vi "运维调试_采配水.vi"() -> ()   [LabVIEW 2016, in "PLC.lvlib"]
uses:
  PLC.lvlib
  <vilib>/Plasmionique/MB Master/MB_Master/MB_Master.lvclass
  <vilib>/Utility/miscctls.llb/LVPointTypeDef.ctl
  <vilib>/Plasmionique/MB Master/MB_Master_Serial/MB_Master_Serial.lvclass
  F:/Program Files/National Instruments/LabVIEW 2016/vi.lib/Plasmionique/MB Master/MB_Master/MB_Master.lvclass
  <vilib>/Plasmionique/MB Master/MB Master.lvlib
panel:
  out "R111":i16 caption="排液时间"
  out "R22":i16
  in  "V8":bool
  out "通讯故障指示":bool
  out "R21":i16
  in  "V7":bool
  out "R20":i16
  in  "M1-2":bool
  in  "潜水泵工作模式":u16(ring) items=["泵1单泵单管路", "泵2单泵单管路", "双泵双管路"]
  out "X10":bool caption="废液报警"
  out "X9":bool caption="自来水报警"
  out "X8":bool caption="泵2过载报警"
  out "X7":bool caption="泵1过载报警"
  out "X6":bool caption="断电检测"
  out "X5":bool caption="开门检测"
  out "X4":bool caption="烟雾检测"
  out "X3":bool caption="漏水检测"
  out "X2":bool caption="进样检测"
  out "X1":bool
  out "X0":bool caption="采样池液位开关"
  out "Y12":bool caption="多参通电"
  out "R109":i16 caption="配水时间"
  out "集成报警信息":string
  out "R108":i16 caption="自来水报警"
  out "R107":i16 caption="采水池液位报警设置"
  out "R106":i16 caption="进样超时设置"
  out "R105":i16 caption="二级清洗时间"
  out "R104":i16 caption="一级清洗时间"
  out "R103":i16 caption="外部管路清洗时间"
  out "R102":i16 caption="静置沉淀时间"
  out "R101":i16 caption="内部管路润洗时间"
  out "R100":i16 caption="外部管路润洗时间"
  out "R2":i16
  out "R1":i16
  out "多列列表框":i32(listbox)
  out "R19":i16
  in  "V6":bool
  out "R18":i16
  in  "V5":bool
  out "R17":i16
  in  "V4":bool
  out "R16":i16
  in  "V3":bool
  out "R15":i16
  in  "V2":bool
  out "R14":i16
  in  "M2":bool
  out "R13":i16
  in  "V1":bool
  out "R12":i16
  in  "M1-1":bool
  in  "返回":bool
  in  "参数设置":bool
  in  "单步启动":bool
  in  "启动":bool
  in  "停止":bool
  # "S"
  # "S"
  # "S"
  # "S"
  # "S"
  # "S"
  # "S"
  # "S"
  # "S"
  # "S"
  # "S"
  # "单步计时："
  # "s"
  # "流程计时："
  # "s"
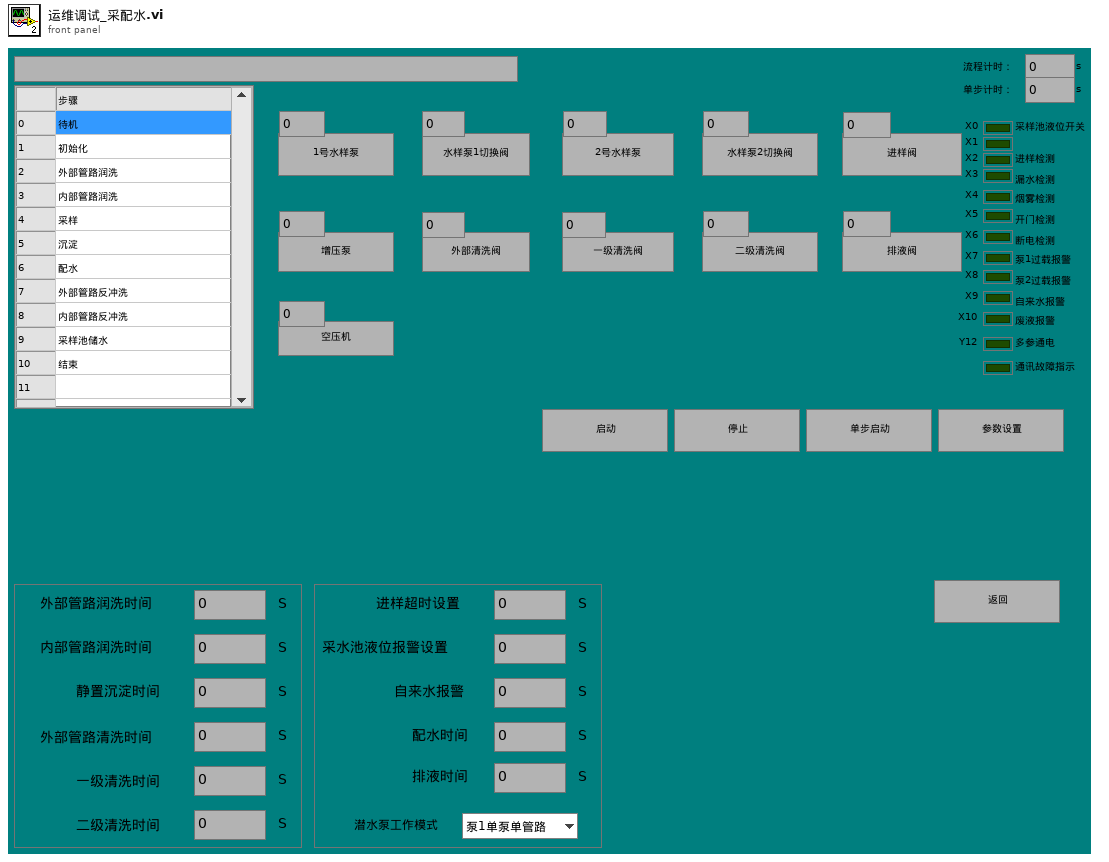
[diagram p1: front panel]
types:
  T1 = typedef "LVPointTypeDef.ctl" = cluster{"Horizontal":i16, "Vertical":i16}
  T2 = cluster{"时间标识":timestamp, "设备":string, "日志信息":string}
  T3 = cluster{"R0":i16, "R1":i16, "R2":i16, "R3":i16, "R4":i16, "R5":i16, "R6":i16, "R7":i16, "R8":i16, "R9":i16, "R10":i16, "R11":i16, "R12":i16, "R13":i16, "R14":i16, "R15":i16, "R16":i16, "R17":i16, "R18":i16, "R19":i16, "R20":i16, "R21":i16, "R22":i16}
  T4 = cluster{"coil values[0]":bool, "coil values[1]":bool, "coil values[2]":bool, "coil values[3]":bool, "coil values[4]":bool, "coil values[5]":bool, "coil values[6]":bool, "coil values[7]":bool, "coil values[8]":bool, "coil values[9]":bool, "coil values[10]":bool, "coil values[11]":bool, "coil values[12]":bool, "coil values[13]":bool, "coil values[14]":bool, "coil values[15]":bool}
  T5 = cluster{"seconds since 1Jan1904":timestamp, "table输入":string, string, "table输入":string}
  T6 = cluster{"时间标识":timestamp, "设备":string, "日志信息":string, "流程参数":string}
  T7 = cluster{"命令":string, cluster{"starting address":u16, "holding register value":u16}}
  T8 = cluster{"CODMn":cluster{"启动测量模式":cluster{"测量模式":enum16{"水样测量", "标样核查", "零点核查", "加标回收", "平行样", "校零", "校标"}}, "确定按钮":bool}, "参数启用":cluster{"多参数":bool, "CODMn":bool, "总磷总氮":bool, "氨氮":bool, "CODcr":bool}}
  T9 = enum16{"水样测量", "标样核查", "零点核查", "加标回收", "平行样", "校零", "校标"}
  T10 = cluster{"命令":string, "数据":cluster{"starting address":u16, "holding register value":u16}}
  T11 = cluster{"命令":string, "数据":cluster{"starting address":u16, "holding register values":u16[]}}
  T12 = cluster{"命令":string, "data":cluster{"starting address":u16, "coil values":bool[]}}
  T13 = enum32{"Bad", "Idle", "Run top level", "Running"}
  T14 = cluster{"baud rate (bps)":u32, "stop bits":u16, "parity":u16, "flow control":u16, "timeout":u32, "retries":i32}
  T15 = cluster{"starting address":u16, "holding register values":u16[]}
  T16 = cluster{"starting address":u16, "holding register value":u16}
  T17 = cluster{"starting address":u16, "coil values":bool[]}
  T18 = cluster{"Registers[0]":u16, "Registers[1]":u16, "Registers[2]":u16, "Registers[3]":u16, "Registers[4]":u16, "Registers[5]":u16, "Registers[6]":u16, "Registers[7]":u16, "Registers[8]":u16, "Registers[9]":u16, "Registers[10]":u16, "Registers[11]":u16, "Registers[12]":u16, "Registers[13]":u16, "Registers[14]":u16, "Registers[15]":u16, "Registers[16]":u16, "Registers[17]":u16, "Registers[18]":u16, "Registers[19]":u16, "Registers[20]":u16, "Registers[21]":u16, "Registers[22]":u16}
  T19 = cluster{"Registers[0]":u16, "Registers[1]":u16, "Registers[2]":u16, "Registers[3]":u16, "Registers[4]":u16, "Registers[5]":u16}
  T20 = cluster{"Coils[0]":bool, "Coils[1]":bool, "Coils[2]":bool, "Coils[3]":bool, "Coils[4]":bool, "Coils[5]":bool, "Coils[6]":bool, "Coils[7]":bool, "Coils[8]":bool, "Coils[9]":bool, "Coils[10]":bool, "Coils[11]":bool, "Coils[12]":bool, "Coils[13]":bool, "Coils[14]":bool, "Coils[15]":bool}
  T21 = cluster{"Registers[0]":u16, "Registers[1]":u16, "Registers[2]":u16, "Registers[3]":u16, "Registers[4]":u16, "Registers[5]":u16, "Registers[6]":u16, "Registers[7]":u16, "Registers[8]":u16, "Registers[9]":u16, "Registers[10]":u16, "Registers[11]":u16, "Registers[12]":u16, "Registers[13]":u16, "Registers[14]":u16, "Registers[15]":u16, "Registers[16]":u16, "Registers[17]":u16, "Registers[18]":u16, "Registers[19]":u16}
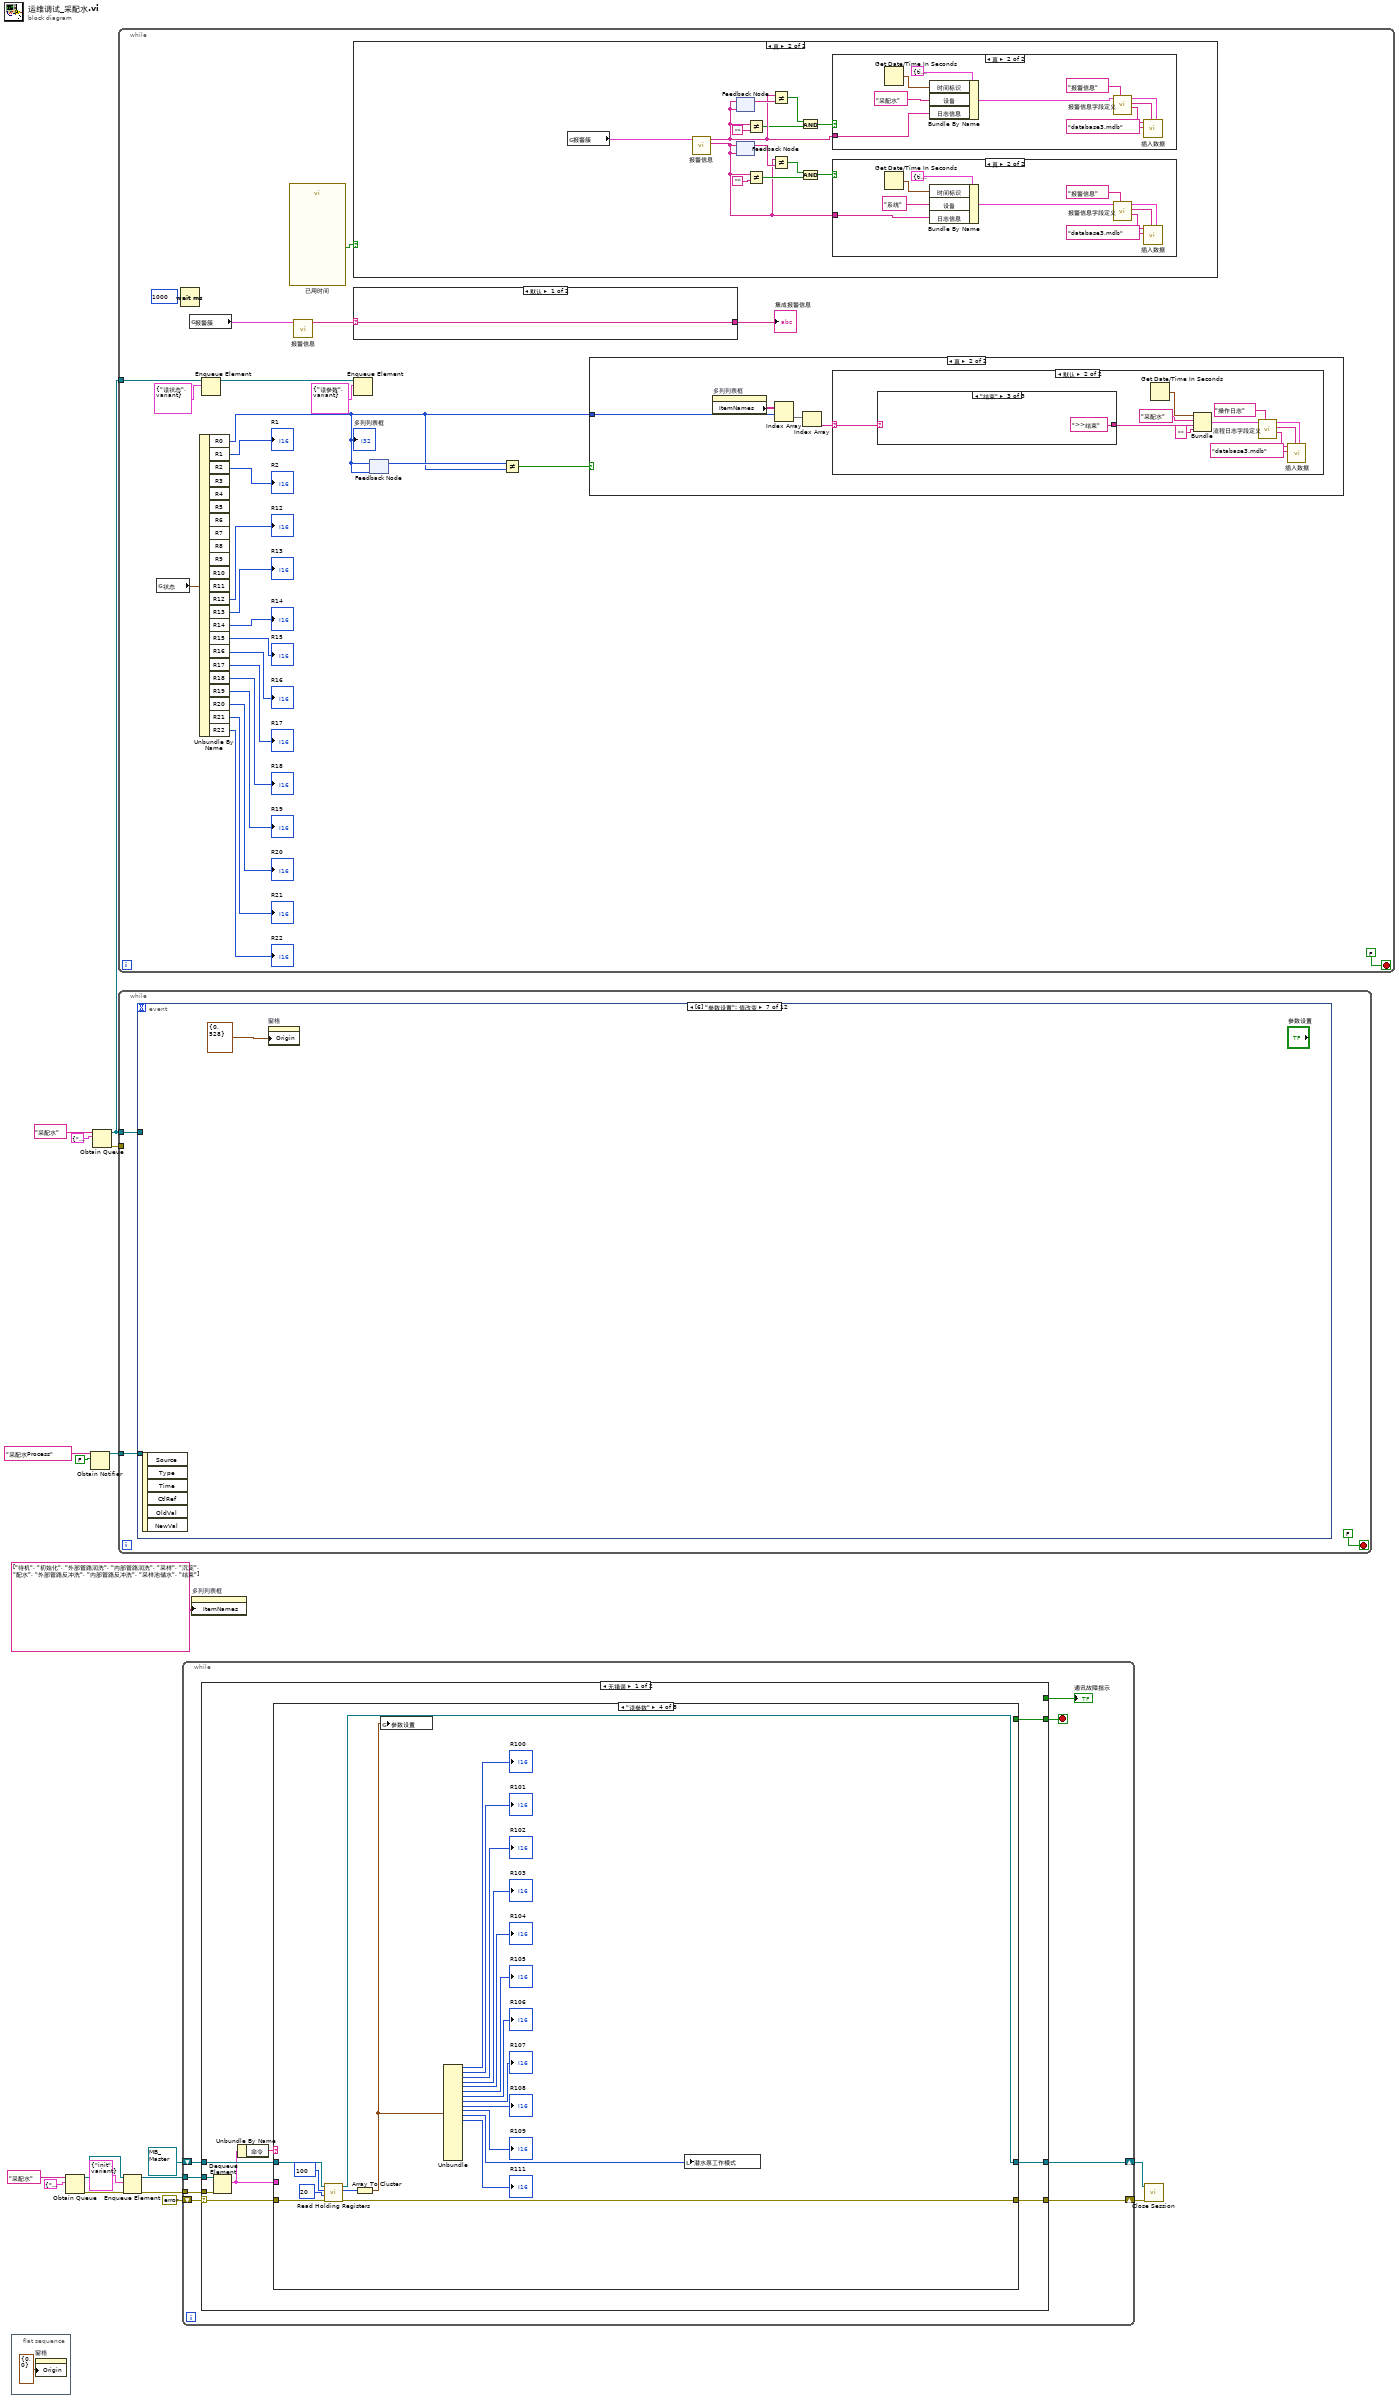
[diagram p0: block diagram]
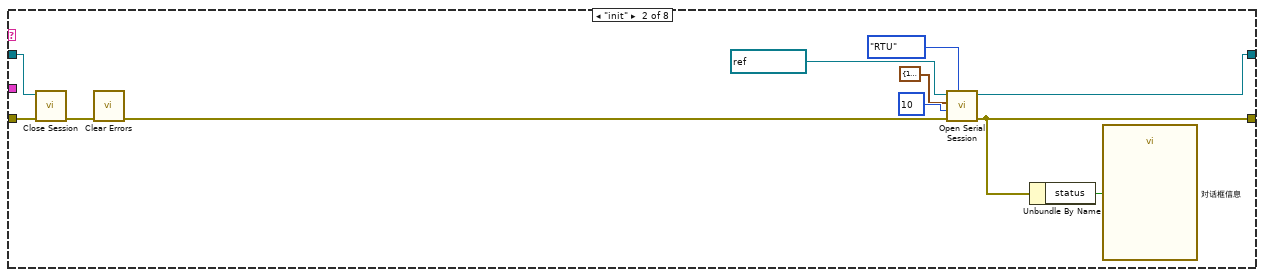
[diagram p3: hidden frame]
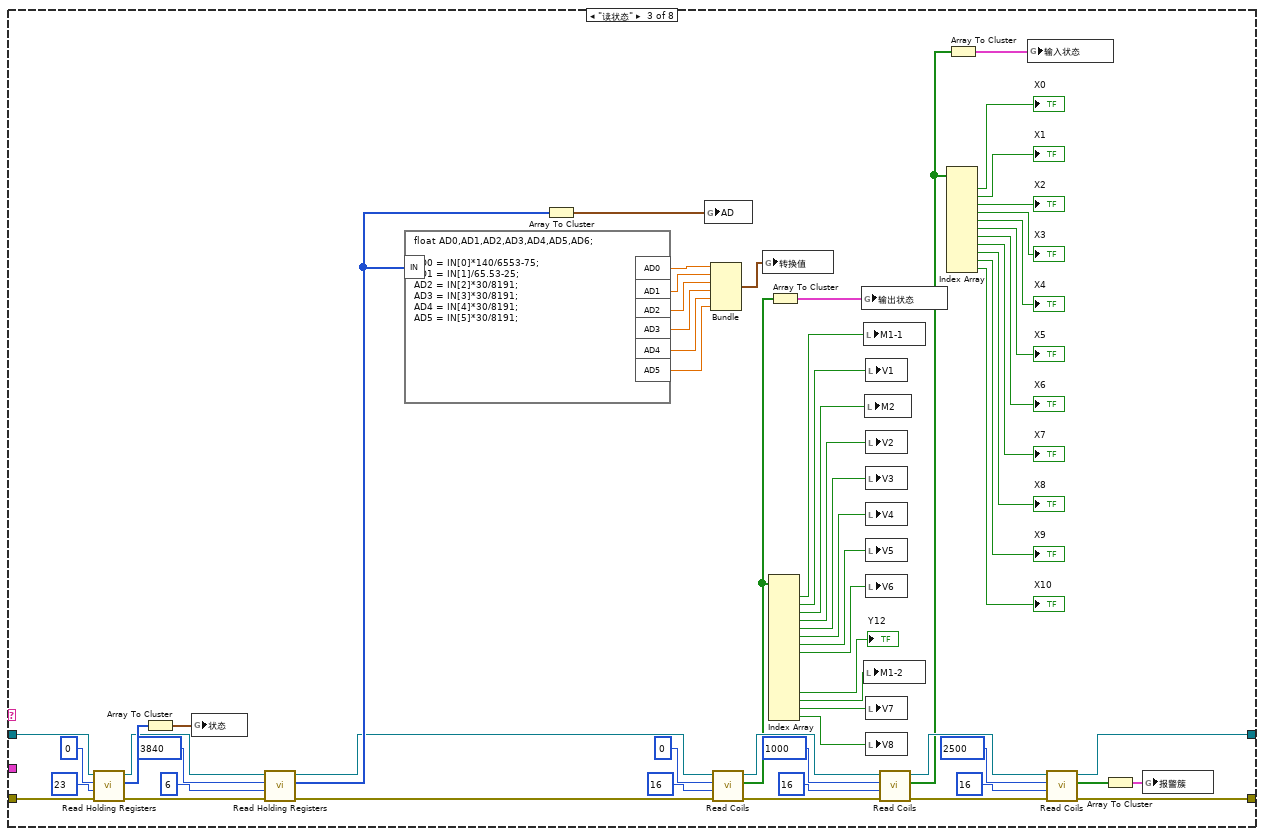
[diagram p4: hidden frame]
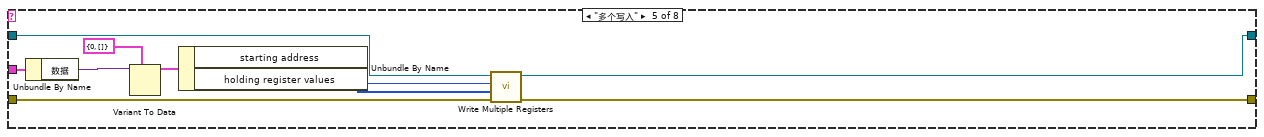
[diagram p5: hidden frame]
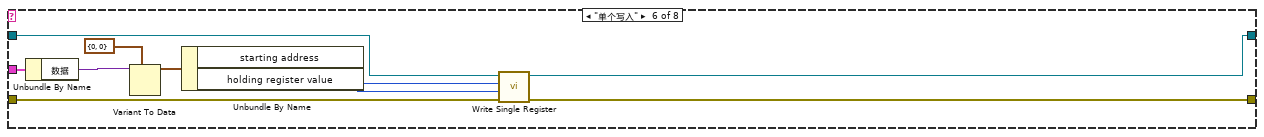
[diagram p6: hidden frame]
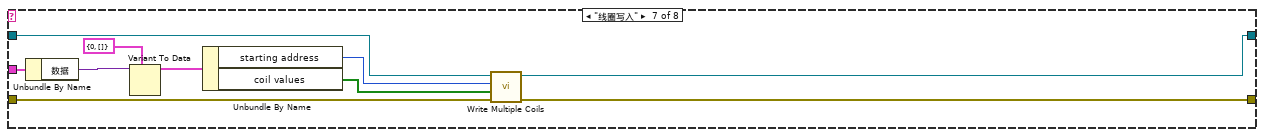
[diagram p7: hidden frame]
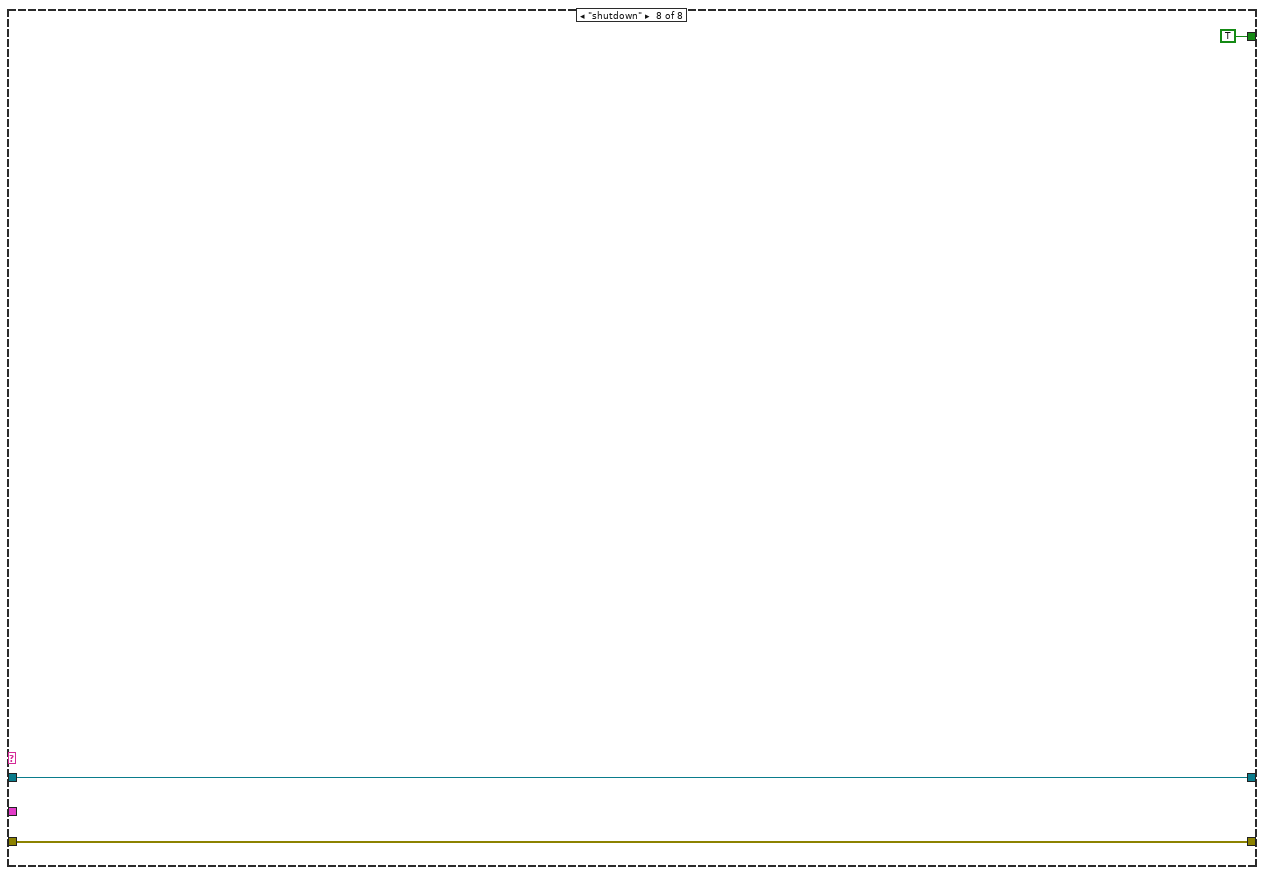
[diagram p8: hidden frame]
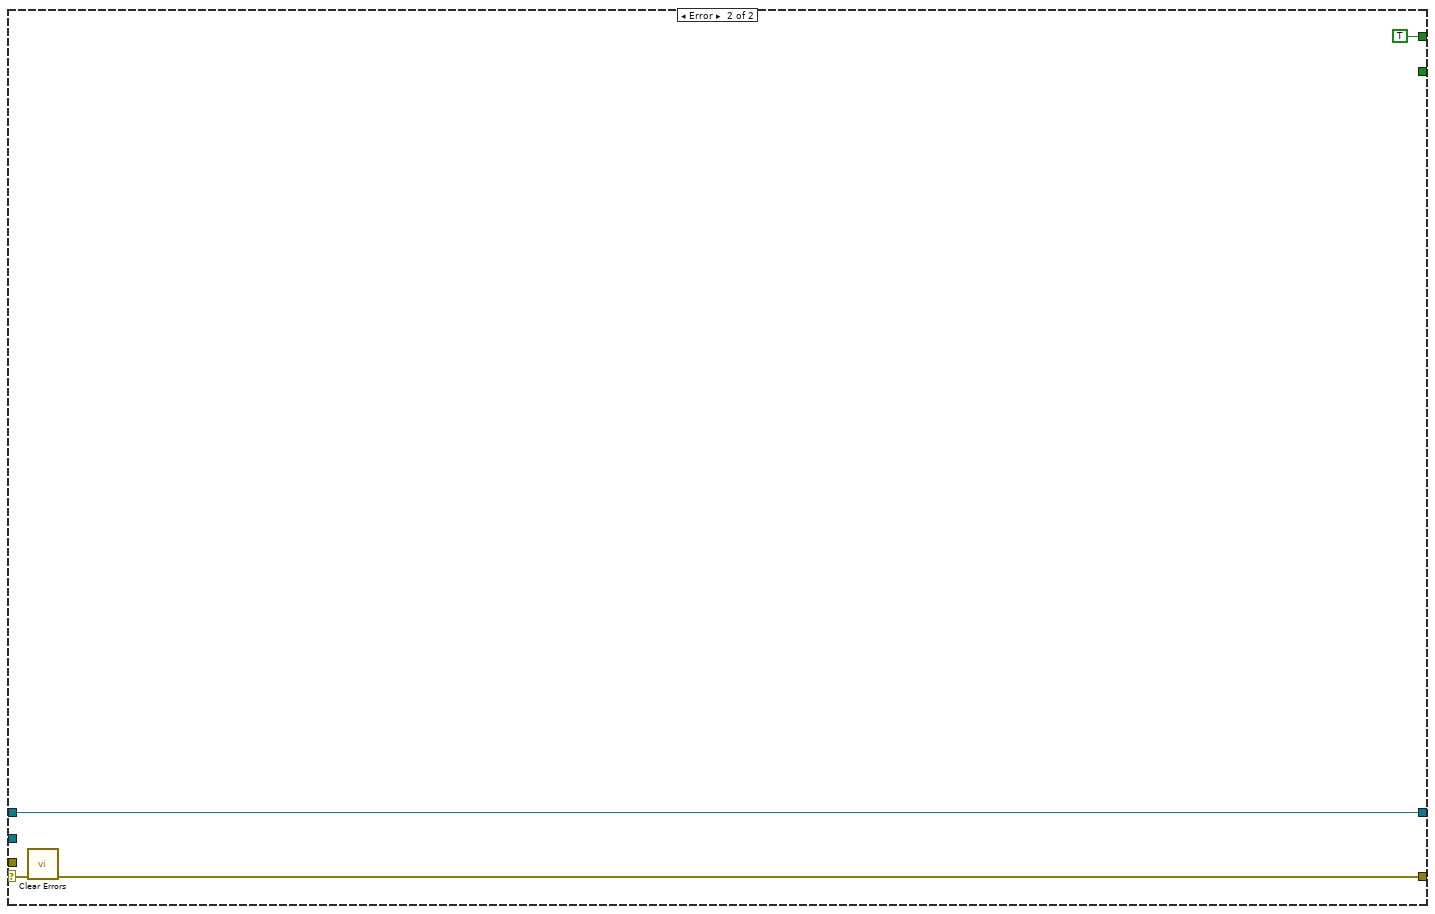
[diagram p9: hidden frame]
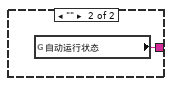
[diagram p13: hidden frame]
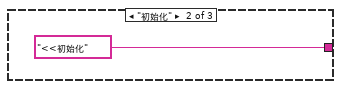
[diagram p17: hidden frame]
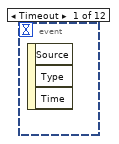
[diagram p18: hidden frame]
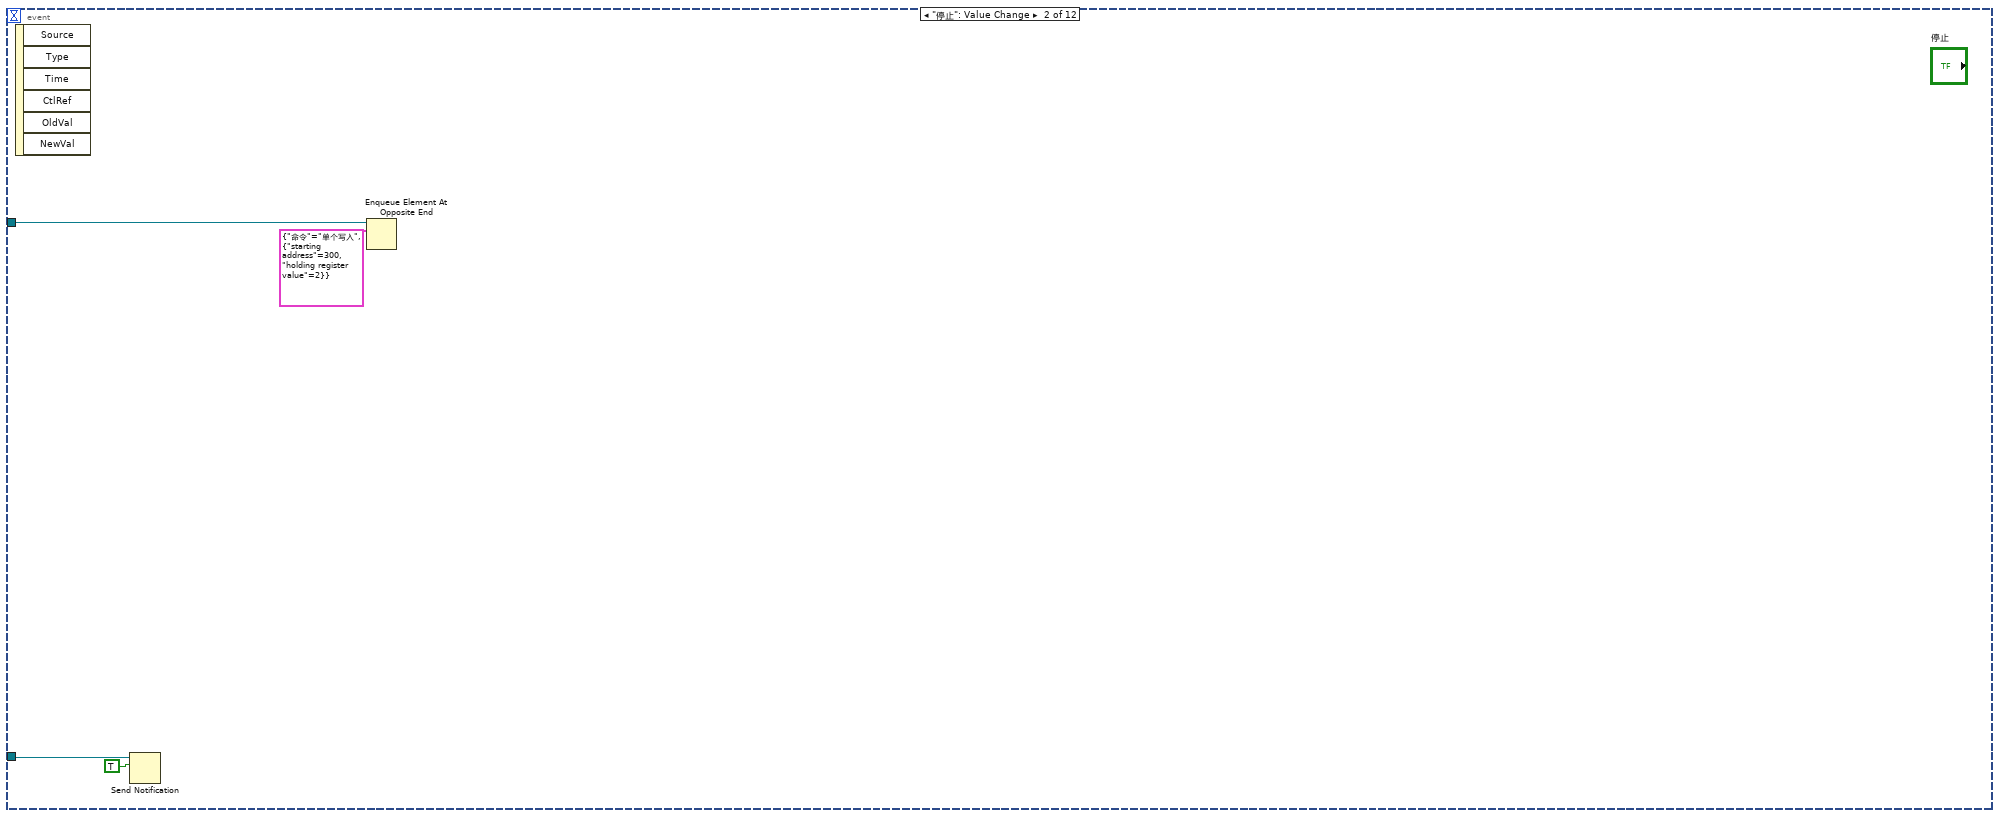
[diagram p19: hidden frame]
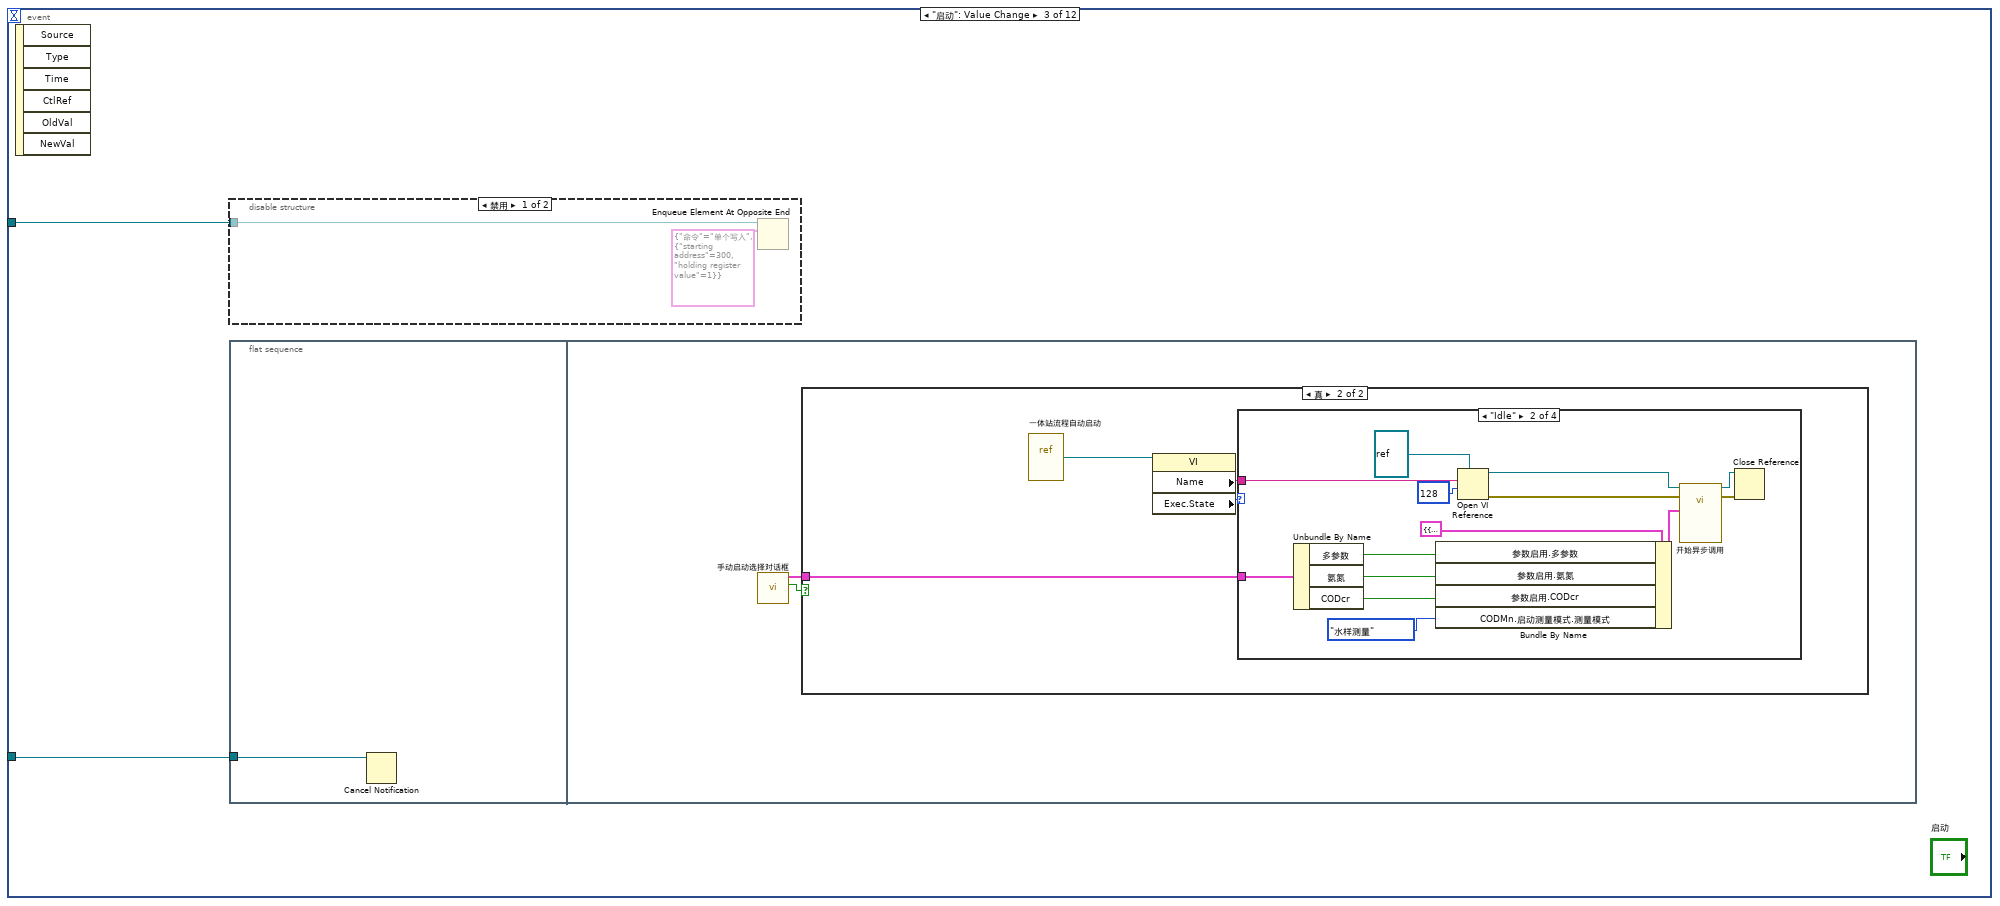
[diagram p20: hidden frame]
diagram:
  n1 = flat-sequence {
    frame #0 {
      n2 = property on="窗格" class="Pane"("Origin"=T1 {"Horizontal"=0, "Vertical"=0} ("原点")) -> ()  [unwired: 2 in, 2 out]
    }
  }
  n3 = Obtain Queue(name (unnamed)="采配水" ("名称（未命名）"), element data type=cluster{"命令":string, "数据":variant} {"命令"="", "数据"=variant}) -> (queue out=w9:refnum<queue>, error out=w8:errorcluster)  [unwired: 3 in, 1 out]
  n4 = Obtain Notifier(name (unnamed)="采配水Process" ("名称（未命名）"), notification data type=FALSE) -> (notifier out=w12:refnum<notifier>)  [unwired: 2 in, 2 out]
  n5 = Obtain Queue(name (unnamed)="采配水" ("名称（未命名）"), element data type=cluster{"命令":string, "数据":variant} {"命令"="", "数据"=variant}) -> (queue out=w16:refnum<queue>, error out=w17:errorcluster)  [unwired: 3 in, 1 out]
  n6 = while {
    tunnel: w16 -> [w46]
    stop <- FALSE stop-if-true
    n7 = global read "采配水全局变量.vi" "状态"() -> (w44:T3)
    n8 = Wait (ms)(milliseconds to wait=u32 1000 ("等待时间（毫秒）")) -> ()  [unwired: 1 out]
    n9 = global read "采配水全局变量.vi" "报警簇"() -> (w32:T4)
    n10 = Unbundle By Name(w44) -> ("R0"=w25:i16, "R1"=→"R1":i16, "R2"=→"R2":i16, "R12"=→"R12":i16, "R13"=→"R13":i16, "R14"=→"R14":i16, "R15"=→"R15":i16, "R16"=→"R16":i16, "R17"=→"R17":i16, "R18"=→"R18":i16, "R19"=→"R19":i16, "R20"=→"R20":i16, "R21"=→"R21":i16, "R22"=→"R22":i16)  [unwired: 9 out]
    "多列列表框" <- w25
    n11 = Enqueue Element(queue=w46, element=cluster{"命令":string, "数据":variant} {"命令"="读状态", "数据"=variant} ("元素")) -> (queue out=w27:refnum<queue>)  [unwired: 2 in, 2 out]
    n12 = call "已用时间"() -> ("Time has Elapsed"=w30:bool)  [unwired: 12 in, 7 out]
    n13 = call "报警信息.vi"("报警簇"=w32) -> ("采配水报警信息"=w24:string)  [unwired: 9 in, 1 out]
    n14 = case shown="真" w30 {
      frame False {
      }
      frame True {
        n15 = global read "采配水全局变量.vi" "报警簇"() -> (w60:T4)
        n16 = call "报警信息.vi"("报警簇"=w60) -> ("系统报警信息"=w49:string, "采配水报警信息"=w56:string)  [unwired: 9 in]
        n17 = feedback #1(w56) -> (w59:string)
        n18 = feedback-in #1(w56) -> ()
        n19 = feedback #2(w49) -> (w50:string)
        n20 = feedback-in #2(w49) -> ()
        n21 = Not Equal?(x=w56, y="") -> (x != y?=w54:bool)
        n22 = Not Equal?(x=w49, y="") -> (x != y?=w53:bool)
        n23 = Not Equal?(x=w56, y=w59) -> (x != y?=w58:bool)
        n24 = Not Equal?(x=w49, y=w50) -> (x != y?=w51:bool)
        n25 = And(x=w58, y=w54) -> (x .and. y?=w57:bool)
        n26 = And(x=w51, y=w53) -> (x .and. y?=w48:bool)
        n27 = case shown="真" w57 {
          tunnel: w56 -> [_ w71]
          frame False {
          }
          frame True {
            n28 = Get Date/Time In Seconds() -> (seconds since 1Jan1904=w73:timestamp)
            n29 = Bundle By Name(cluster=T2 {"时间标识"=timestamp(0 s since 1904-01-01), "设备"="", "日志信息"=""} ("data in"), "时间标识"=w73, "设备"="采配水", "日志信息"=w71) -> (w74:T2)
            n30 = call "报警信息字段定义.vi"("table输入"="报警信息", "data in"=w74) -> ("table输出"=w78:string, "columns"=w79:string[], "data out"=w80:T2)  [unwired: 7 in]
            n31 = call "插入数据.vi"("data"=w80, "columns"=w79, "database"="database3.mdb", "table"=w78) -> ()  [unwired: 7 in, 1 out]
          }
        }
        n32 = case shown="真" w48 {
          tunnel: w49 -> [_ w61]
          frame False {
          }
          frame True {
            n33 = Get Date/Time In Seconds() -> (seconds since 1Jan1904=w63:timestamp)
            n34 = Bundle By Name(cluster=T2 {"时间标识"=timestamp(0 s since 1904-01-01), "设备"="", "日志信息"=""} ("data in"), "时间标识"=w63, "设备"="系统", "日志信息"=w61) -> (w64:T2)
            n35 = call "报警信息字段定义.vi"("table输入"="报警信息", "data in"=w64) -> ("table输出"=w68:string, "columns"=w69:string[], "data out"=w70:T2)  [unwired: 7 in]
            n36 = call "插入数据.vi"("data"=w70, "columns"=w69, "database"="database3.mdb", "table"=w68) -> ()  [unwired: 7 in, 1 out]
          }
        }
      }
    }
    n37 = case shown="默认" w24 {
      selector: w24 -> [w81 _]
      tunnel: [w81 w82] -> w31
      frame Default {
      }
      frame "" {
        n38 = global read "采配水全局变量.vi" "自动运行状态"() -> (w82:string)
      }
    }
    "集成报警信息" <- w31
    n39 = Enqueue Element(queue=w27, element=cluster{"命令":string, "数据":variant} {"命令"="读参数", "数据"=variant} ("元素")) -> ()  [unwired: 2 in, 3 out]
    n40 = feedback-in #3(w25) -> ()
    n41 = feedback #3(w25) -> (w26:i16)
    n42 = Not Equal?(x=w26, y=w25) -> (x != y?=w33:bool)
    n43 = case shown="真" w33 {
      tunnel: w25 -> [_ w85]
      frame False {
      }
      frame True {
        n44 = property on="多列列表框" class="MCListbox (严格)"() -> ("ItemNames"=w86:string[][])  [unwired: 2 in, 2 out]
        n45 = Index Array(array=w86, index (row)=w85) -> (element=w84:string[])  [unwired: 1 in]
        n46 = Index Array(array=w84) -> (element=w83:string)  [unwired: 1 in]
        n47 = case shown="默认" w83 {
          selector: w83 -> [_ w88]
          frame "待机" {
          }
          frame Default {
            n48 = case shown="\"结束\"" w88 {
              selector: w88 -> [w98 _ _]
              tunnel: [w98 "<<初始化" ">>结束"] -> w87
              frame Default {
              }
              frame "初始化" {
              }
              frame "结束" {
              }
            }
            n49 = Get Date/Time In Seconds() -> (seconds since 1Jan1904=w92:timestamp)
            n50 = Bundle("seconds since 1Jan1904"=w92, "table输入"="采配水", w87, "table输入"="") -> (w90:T5)  [unwired: 1 in]
            n51 = call "流程日志字段定义.vi"("table输入"="操作日志", "data in"=w90) -> ("table输出"=w95:string, "columns"=w96:string[], "data out"=w97:T6)  [unwired: 7 in]
            n52 = call "插入数据.vi"("data"=w97, "columns"=w96, "database"="database3.mdb", "table"=w95) -> ()  [unwired: 7 in, 1 out]
          }
        }
      }
    }
  }
  n53 = while {
    tunnel: w16 -> [w102]
    tunnel: w17 -> [_]
    tunnel: w12 -> [w101]
    stop <- FALSE stop-if-true
    n54 = event shown="[6] \"参数设置\": 值改变" {
      selector: _ -> [_ _ _ _ _ _ _ _ _ _ _ _]
      dyn-events: _ -> [_ _ _ _ _ _ _ _ _ _ _ _]
      timeout: _ -> [_ _ _ _ _ _ _ _ _ _ _ _]
      tunnel: w102 -> [_ w106 w109 w137 w154 _ _ _ w172 w174 w179 w184]
      tunnel: w101 -> [_ w105 w108 _ _ _ _ _ _ _ _ _]
      event Timeout {
        n55 = event-data() -> ()  [unwired: 1 in, 3 out]
      }
      event "停止": Value Change {
        n56 = event-data() -> ()  [unwired: 1 in, 6 out]
        n57 = Send Notification(notification=TRUE ("通知"), notifier=w105) -> ()  [unwired: 1 in, 2 out]
        n58 = Enqueue Element At Opposite End(queue=w106, element=T7 {"命令"="单个写入", {"starting address"=300, "holding register value"=2}} ("元素")) -> ()  [unwired: 2 in, 3 out]
      }
      event "启动": Value Change {
        n59 = event-data() -> ()  [unwired: 1 in, 6 out]
        n60 = disable-structure shown="禁用" {
          disable-tunnel: w109 -> [w133 _]
          frame Disabled {
            n61 = Enqueue Element At Opposite End(queue=w133, element=T7 {"命令"="单个写入", {"starting address"=300, "holding register value"=1}} ("元素")) -> ()  [unwired: 2 in, 3 out]
          }
          frame Enabled {
          }
        }
        n62 = flat-sequence {
          tunnel: w108 -> [w110]
          frame #0 {
            n63 = Cancel Notification(0:w110) -> ()  [unwired: 1 in, 3 out]
          }
          frame #1 {
            n64 = call "手动启动选择对话框.vi"() -> ("确定"=w112:bool, "输出簇"=w111:cluster{"多参数":bool, "氨氮":bool, "CODcr":bool})  [unwired: 10 in]
            n65 = case shown="真" w112 {
              tunnel: w111 -> [_ w113]
              frame False {
              }
              frame True {
                n66 = vi-ref "一体站流程自动启动.vi"() -> (w116:refnum<vi>)
                n67 = property class="VI"(reference=w116) -> ("Name"=w115:string, "Exec.State"=w114:T13)  [unwired: 1 in, 2 out]
                n68 = case shown="\"Idle\"" w114 {
                  tunnel: w115 -> [_ w130 _ _]
                  tunnel: w113 -> [_ w120 _ _]
                  frame "Bad", Default {
                  }
                  frame "Idle" {
                    n69 = Unbundle By Name(w120) -> ("多参数"=w119:bool, "氨氮"=w118:bool, "CODcr"=w117:bool)
                    n70 = Bundle By Name(cluster=T8 {"CODMn"={"启动测量模式"={"测量模式"=enum."水样测量"}, "确定按钮"=FALSE}, "参数启用"={"多参数"=FALSE, "CODMn"=FALSE, "总磷总氮"=FALSE, "氨氮"=FALSE, "CODcr"=FALSE}} ("参数"), "参数启用.多参数"=w119, "参数启用.氨氮"=w118, "参数启用.CODcr"=w117, "CODMn.启动测量模式.测量模式"=T9."水样测量") -> (w121:T8)
                    n71 = Open VI Reference(type specifier VI Refnum (for type only)=refnum<vi> refnum, vi path=w130, options=128 ("选项")) -> (vi reference=w128:refnum<vi>, error out=w125:errorcluster)  [unwired: 3 in]
                    n72 = call-by-ref "开始异步调用"(reference=w128, error in=w125, "参数"=w121) -> (reference out=w126:refnum<vi>, error out=w124:errorcluster)  [unwired: 11 in]
                    n73 = Close Reference(reference=w126, error in (no error)=w124) -> ()  [unwired: 1 out]
                  }
                  frame "Run top level" {
                  }
                  frame "Running" {
                    n74 = One Button Dialog(message="流程已经运行,无须重复启动" ("消息")) -> ()  [unwired: 1 in, 1 out]
                  }
                }
              }
            }
          }
        }
      }
      event "单步启动": Value Change {
        n75 = event-data() -> ()  [unwired: 1 in, 6 out]
        n76 = call "单步启动对话框.vi"() -> ("单步启动步骤输出"=w134:u16)  [unwired: 11 in]
        n77 = Bundle By Name(cluster=T10 {"命令"="单个写入", "数据"={"starting address"=301, "holding register value"=0}} ("元素"), "数据.holding register value"=w134) -> (w135:T10)
        n78 = Enqueue Element At Opposite End(queue=w137, element=w135) -> ()  [unwired: 2 in, 3 out]
      }
      event "R100", "R101", "R102", "R103", "R104", "R105", "R106", "R107", "R108", "R109", "潜水泵工作模式": Value Change {
        n79 = event-data() -> ()  [unwired: 1 in, 6 out]
        n80 = local read "R100"() -> (w149:i16)
        n81 = local read "R101"() -> (w148:i16)
        n82 = local read "R102"() -> (w147:i16)
        n83 = local read "R103"() -> (w146:i16)
        n84 = local read "R104"() -> (w145:i16)
        n85 = local read "R105"() -> (w144:i16)
        n86 = local read "R106"() -> (w143:i16)
        n87 = local read "R107"() -> (w142:i16)
        n88 = local read "R108"() -> (w141:i16)
        n89 = local read "R109"() -> (w140:i16)
        n90 = local read "R111"() -> (w138:i16)
        n91 = Build Array(w149, w148, w147, w146, w145, w144, w143, w142, w141, w140, "潜水泵工作模式", w138) -> (w150:u16[])
        n92 = Bundle By Name(cluster=T11 {"命令"="多个写入", "数据"={"starting address"=0, "holding register values"=[]}} ("元素"), "数据.starting address"=u16 100, "数据.holding register values"=w150) -> (w151:T11)
        n93 = Enqueue Element At Opposite End(queue=w154, element=w151) -> ()  [unwired: 2 in, 3 out]
      }
      event "R100", "R101", "R102", "R103", "R104", "R105", "R106", "R107", "R108", "R109", "R111": Mouse Down {
        n94 = event-data() -> ("CtlRef"=w158:refnum<vi>)  [unwired: 1 in, 7 out]
        n95 = property class="DigNum (严格)"(reference=w158) -> (reference out=w156:refnum<vi>, "Value"=w157:i16)  [unwired: 1 in, 1 out]
        n96 = call "数字键盘.vi"("OldNumber"=w157) -> ("NewNumber"=w155:sgl)
        n97 = property class="DigNum (严格)"(reference=w156, "Val(Sgnl)"=w155) -> ()  [unwired: 1 in, 2 out]
      }
      event "参数设置": Value Change {
        n98 = event-data() -> ()  [unwired: 1 in, 6 out]
        n99 = property on="窗格" class="Pane"("Origin"=T1 {"Horizontal"=0, "Vertical"=528} ("原点")) -> ()  [unwired: 2 in, 2 out]
      }
      event "返回": Value Change {
        n100 = event-data() -> ()  [unwired: 1 in, 6 out]
        n101 = property on="窗格" class="Pane"("Origin"=T1 {"Horizontal"=0, "Vertical"=0} ("原点")) -> ()  [unwired: 2 in, 2 out]
      }
      event "M1-1", "V1", "M2", "V2", "V3", "V4", "V5", "V6": Value Change {
        n102 = event-data() -> ()  [unwired: 1 in, 6 out]
        n103 = Build Array("M1-1", "V1", "M2", "V2", "V3", "V4", "V5", "V6") -> (w161:bool[])
        n104 = Bundle By Name(cluster=T12 {"命令"="线圈写入", "data"={"starting address"=2400, "coil values"=[]}} ("元素"), "data.coil values"=w161) -> (w162:T12)
        n105 = Enqueue Element(queue=w172, element=w162) -> ()  [unwired: 2 in, 3 out]
      }
      event "M1-2": Value Change {
        n106 = event-data() -> ()  [unwired: 1 in, 6 out]
        n107 = Build Array("M1-2") -> (w175:bool[])
        n108 = Bundle By Name(cluster=T12 {"命令"="线圈写入", "data"={"starting address"=2413, "coil values"=[]}} ("元素"), "data.coil values"=w175) -> (w176:T12)
        n109 = Enqueue Element(queue=w174, element=w176) -> ()  [unwired: 2 in, 3 out]
      }
      event "V7": Value Change {
        n110 = event-data() -> ()  [unwired: 1 in, 6 out]
        n111 = Build Array("V7") -> (w180:bool[])
        n112 = Bundle By Name(cluster=T12 {"命令"="线圈写入", "data"={"starting address"=2414, "coil values"=[]}} ("元素"), "data.coil values"=w180) -> (w181:T12)
        n113 = Enqueue Element(queue=w179, element=w181) -> ()  [unwired: 2 in, 3 out]
      }
      event "V8": Value Change {
        n114 = event-data() -> ()  [unwired: 1 in, 6 out]
        n115 = Build Array("V8") -> (w185:bool[])
        n116 = Bundle By Name(cluster=T12 {"命令"="线圈写入", "data"={"starting address"=2415, "coil values"=[]}} ("元素"), "data.coil values"=w185) -> (w186:T12)
        n117 = Enqueue Element(queue=w184, element=w186) -> ()  [unwired: 2 in, 3 out]
      }
    }
  }
  n118 = Enqueue Element(queue=w9, element=cluster{"命令":string, "数据":variant} {"命令"="init", "数据"=variant} ("元素"), error in (no error)=w8) -> (queue out=w5:refnum<queue>, error out=w6:errorcluster)  [unwired: 1 in, 1 out]
  n119 = while {
    tunnel: w5 -> [w192]
    tunnel: w6 -> [w191]
    shift-right: [w195] -> w2
    shift-left: refnum<class "MB_Master.lvclass"> refnum ("MB session in") -> [w194]
    shift-right: [w193] -> w3
    shift-left: errorcluster {"status"=FALSE, "code"=0, "source"=""} ("error out") -> [w189]
    stop <- w190 stop-if-true
    n120 = case shown="无错误" w189 {
      selector: w189 -> [w201 w336]
      tunnel: [w204 w334] -> w195
      tunnel: w194 -> [w203 w334]
      tunnel: [w202 w335] -> w193
      tunnel: w192 -> [w198 _]
      tunnel: w191 -> [w197 _]
      tunnel: [w199 _] -> w190
      tunnel: [_ TRUE ("通讯故障指示")] -> w188
      frame No Error {
        n121 = Dequeue Element(queue=w198, error in (no error)=w197) -> (element=w196:cluster{"命令":string, "数据":variant})  [unwired: 1 in, 3 out]
        n122 = Unbundle By Name(w196) -> ("命令"=w200:string)
        n123 = case shown="\"读参数\"" w200 {
          tunnel: [w206 w207 w244 w294 w306 w316 w326 w331] -> w204
          tunnel: w203 -> [w206 w214 w264 w299 w309 w319 w329 w331]
          tunnel: [w205 w212 w243 w293 w307 w317 w327 w330] -> w202
          tunnel: w201 -> [w205 w216 w267 w298 w308 w318 w328 w330]
          tunnel: [_ _ _ _ _ _ _ TRUE] -> w199
          tunnel: w196 -> [_ _ _ _ w305 w315 w325 _]
          frame "idle", Default {
          }
          frame "init" {
            n124 = call-dynamic "Close Session.vi"("error in (no error)"=w216, "MB session in"=w214) -> ("error out"=w215:errorcluster)  [unwired: 9 in]
            n125 = call <vilib>:"Clear Errors.vi"("error in (no error)"=w215) -> ("error out"=w213:errorcluster)  [unwired: 5 in, 1 out]
            n126 = call <vilib>:"Open Serial Session.vi"("Mode (RTU)"=enum16{"RTU", "ASCII"}."RTU", "Error in"=w213, "Slave ID"=u8 10, "Serial Config"=T14 {"baud rate (bps)"=115200, "stop bits"=10, "parity"=0, "flow control"=0, "timeout"=100, "retries"=1}, "VISA Resource"=refnum<visa-resource-name> "COM2" ("VISA resource name")) -> ("Error out"=w212:errorcluster, "MB_Serial session"=w207:refnum<class "MB_Master_Serial.lvclass">)  [unwired: 5 in]
            n127 = Unbundle By Name(w212) -> ("status"=w217:bool)
            n128 = call "对话框信息"("Enable"=w217) -> ()  [unwired: 9 in, 2 out]
          }
          frame "读状态" {
            n129 = call <vilib>:"Read Holding Registers.vi"("error in (no error)"=w267, "quantity"=u16 23 ("number of holding registers"), "starting address"=u16 0, "MB session in"=w264) -> ("error out"=w260:errorcluster, "Registers"=w263:u16[], "MB session out"=w262:refnum<class "MB_Master.lvclass">)  [unwired: 5 in]
            n130 = Array To Cluster(array=w263) -> (cluster=w269:T18)
            n131 = global write "采配水全局变量.vi" "状态"(w269) -> ()
            n132 = call <vilib>:"Read Holding Registers.vi"("error in (no error)"=w260, "quantity"=u16 6 ("number of holding registers"), "starting address"=u16 3840, "MB session in"=w262) -> ("error out"=w256:errorcluster, "Registers"=w261:u16[], "MB session out"=w257:refnum<class "MB_Master.lvclass">)  [unwired: 5 in]
            n133 = formula code="float AD0,AD1,AD2,AD3,AD4,AD5,AD6;\n\nAD0 = IN[0]*140/6553-75;\nAD1 = IN[1]/65.53-25;\nAD2 = IN[2]*30/8191;\nAD3 = IN[3]*30/8191;\nAD4 = IN[4]*30/8191;\nAD5 = IN[5]*30/8191;"("IN"=w261) -> ("AD0"=w275:dbl, "AD1"=w274:dbl, "AD2"=w273:dbl, "AD3"=w272:dbl, "AD4"=w271:dbl, "AD5"=w270:dbl)
            n134 = Array To Cluster(array=w261) -> (cluster=w277:T19)
            n135 = global write "采配水全局变量.vi" "AD"(w277) -> ()
            n136 = Bundle(w275, w274, w273, w272, w271, w270) -> (w276:cluster{dbl, dbl, dbl, dbl, dbl, dbl})  [unwired: 1 in]
            n137 = call <vilib>:"Read Coils.vi"("error in (no error)"=w256, "quantity"=u16 16 ("number of coils"), "starting address"=u16 0, "MB session in"=w257) -> ("error out"=w252:errorcluster, "Coils"=w233:bool[], "MB session out"=w253:refnum<class "MB_Master.lvclass">)  [unwired: 5 in]
            n138 = global write "采配水全局变量.vi" "转换值"(w276) -> ()
            n139 = Index Array(array=w233) -> (element #1=w228:bool, element #2=w227:bool, element #3=w226:bool, element #4=w225:bool, element #5=w224:bool, element #6=w223:bool, element #7=w222:bool, element #8=w221:bool, element #13=→"Y12":bool, element #14=w220:bool, element #15=w219:bool, element #16=w218:bool)  [unwired: 16 in, 4 out]
            n140 = Array To Cluster(array=w233) -> (cluster=w278:T20)
            n141 = global write "采配水全局变量.vi" "输出状态"(w278) -> ()
            n142 = local write "M1-1"(w228) -> ()
            n143 = local write "M1-2"(w220) -> ()
            n144 = local write "M2"(w226) -> ()
            n145 = local write "V1"(w227) -> ()
            n146 = local write "V2"(w225) -> ()
            n147 = local write "V3"(w224) -> ()
            n148 = local write "V4"(w223) -> ()
            n149 = local write "V5"(w222) -> ()
            n150 = local write "V6"(w221) -> ()
            n151 = local write "V7"(w219) -> ()
            n152 = local write "V8"(w218) -> ()
            n153 = call <vilib>:"Read Coils.vi"("error in (no error)"=w252, "quantity"=u16 16 ("number of coils"), "starting address"=u16 1000, "MB session in"=w253) -> ("error out"=w248:errorcluster, "Coils"=w242:bool[], "MB session out"=w249:refnum<class "MB_Master.lvclass">)  [unwired: 5 in]
            n154 = Index Array(array=w242) -> (element #1=→"X0":bool, element #2=→"X1":bool, element #3=→"X2":bool, element #4=→"X3":bool, element #5=→"X4":bool, element #6=→"X5":bool, element #7=→"X6":bool, element #8=→"X7":bool, element #9=→"X8":bool, element #10=→"X9":bool, element #11=→"X10":bool)  [unwired: 11 in]
            n155 = Array To Cluster(array=w242) -> (cluster=w279:T20)
            n156 = global write "采配水全局变量.vi" "输入状态"(w279) -> ()
            n157 = call <vilib>:"Read Coils.vi"("error in (no error)"=w248, "quantity"=u16 16 ("number of coils"), "starting address"=u16 2500, "MB session in"=w249) -> ("error out"=w243:errorcluster, "Coils"=w245:bool[], "MB session out"=w244:refnum<class "MB_Master.lvclass">)  [unwired: 5 in]
            n158 = Array To Cluster(array=w245) -> (cluster=w268:T20)
            n159 = global write "采配水全局变量.vi" "报警簇"(w268) -> ()
          }
          frame "读参数" {
            n160 = call <vilib>:"Read Holding Registers.vi"("error in (no error)"=w298, "quantity"=u16 20 ("number of holding registers"), "starting address"=u16 100, "MB session in"=w299) -> ("error out"=w293:errorcluster, "Registers"=w295:u16[], "MB session out"=w294:refnum<class "MB_Master.lvclass">)  [unwired: 5 in]
            n161 = Array To Cluster(array=w295) -> (cluster=w282:T21)
            n162 = global write "采配水全局变量.vi" "参数设置"(w282) -> ()
            n163 = Unbundle(w282) -> ("Registers[0]"=→"R100":u16, "Registers[1]"=→"R101":u16, "Registers[2]"=→"R102":u16, "Registers[3]"=→"R103":u16, "Registers[4]"=→"R104":u16, "Registers[5]"=→"R105":u16, "Registers[6]"=→"R106":u16, "Registers[7]"=→"R107":u16, "Registers[8]"=→"R108":u16, "Registers[9]"=→"R109":u16, "Registers[10]"=w281:u16, "Registers[11]"=→"R111":u16)  [unwired: 8 out]
            n164 = local write "潜水泵工作模式"(w281) -> ()
          }
          frame "多个写入" {
            n165 = Unbundle By Name(w305) -> ("数据"=w304:variant)
            n166 = Variant To Data(type=T15 {"starting address"=0, "holding register values"=[]}, Variant=w304) -> (data=w302:T15)  [unwired: 1 in, 1 out]
            n167 = Unbundle By Name(w302) -> ("starting address"=w301:u16, "holding register values"=w300:u16[])
            n168 = call <vilib>:"Write Multiple Registers.vi"("error in (no error)"=w308, "values"=w300, "starting address"=w301, "MB session in"=w309) -> ("error out"=w307:errorcluster, "MB session out"=w306:refnum<class "MB_Master.lvclass">)  [unwired: 6 in]
          }
          frame "单个写入" {
            n169 = Unbundle By Name(w315) -> ("数据"=w314:variant)
            n170 = Variant To Data(type=T16 {"starting address"=0, "holding register value"=0}, Variant=w314) -> (data=w312:T16)  [unwired: 1 in, 1 out]
            n171 = Unbundle By Name(w312) -> ("starting address"=w311:u16, "holding register value"=w310:u16)
            n172 = call <vilib>:"Write Single Register.vi"("error in (no error)"=w318, "value"=w310, "address"=w311, "MB session in"=w319) -> ("error out"=w317:errorcluster, "MB session out"=w316:refnum<class "MB_Master.lvclass">)  [unwired: 6 in]
          }
          frame "线圈写入" {
            n173 = Unbundle By Name(w325) -> ("数据"=w324:variant)
            n174 = Variant To Data(type=T17 {"starting address"=0, "coil values"=[]}, Variant=w324) -> (data=w322:T17)  [unwired: 1 in, 1 out]
            n175 = Unbundle By Name(w322) -> ("starting address"=w321:u16, "coil values"=w320:bool[])
            n176 = call <vilib>:"Write Multiple Coils.vi"("error in (no error)"=w328, "values"=w320, "starting address"=w321, "MB session in"=w329) -> ("error out"=w327:errorcluster, "MB session out"=w326:refnum<class "MB_Master.lvclass">)  [unwired: 6 in]
          }
          frame "shutdown" {
          }
        }
      }
      frame Error {
        n177 = call <vilib>:"Clear Errors.vi"("error in (no error)"=w336) -> ("error out"=w335:errorcluster)  [unwired: 5 in, 1 out]
      }
    }
    "通讯故障指示" <- w188
  }
  n178 = property on="多列列表框" class="MCListbox (严格)"("ItemNames"=string[][] [["待机"], ["初始化"], ["外部管路润洗"], ["内部管路润洗"], ["采样"], ["沉淀"], ["配水"], ["外部管路反冲洗"], ["内部管路反冲洗"], ["采样池储水"], ["结束"]] ("项名")) -> ()  [unwired: 2 in, 2 out]
  n179 = call-dynamic "Close Session.vi"("error in (no error)"=w3, "MB session in"=w2) -> ()  [unwired: 9 in, 1 out]
